vi "Edit IPI Dialog.vi"(8 "Coords":T1, 11 "Expr In":string) -> (3 "Expr Out":string)   [LabVIEW 2020]
uses:
  <vilib>/Utility/miscctls.llb/LVPoint32TypeDef.ctl
  epl-vi-lib/Utility VIs/Error Handling VIs/Error-Library Action.ctl
panel:
  in  "Tab Control":enum32{"Hist", "Error"}(tab)
  out "histogram":cluster{"X/1000":dbl[], "Y":dbl[]}(graph)
  out "Message":string
  out "replot":bool
  in  "Expr":string
  in  "Cancel":bool
  in  "OK":bool
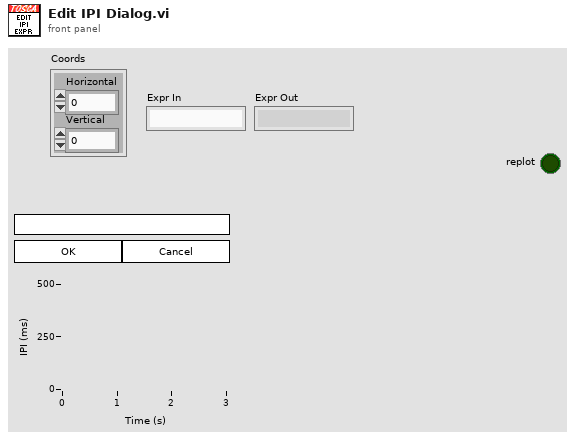
[diagram p1: front panel]
types:
  T1 = typedef "LVPoint32TypeDef.ctl" = cluster{"Horizontal":i32, "Vertical":i32}
  T2 = typedef "Error-Library Action.ctl" = enum16{"NONE", "Register", "Read"}
  T3 = typedef "Error Description.ctl" = cluster{"Code":i32, "Description":string, "Details":string}
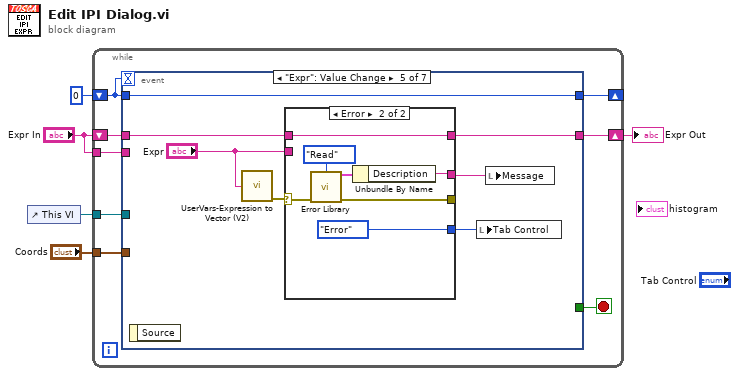
[diagram p0: block diagram]
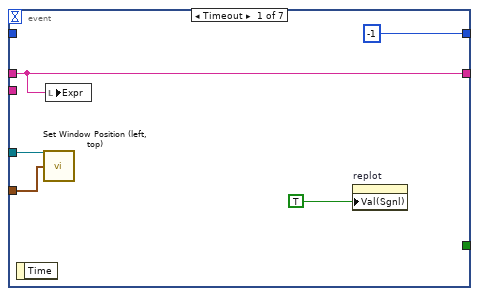
[diagram p2: hidden frame]
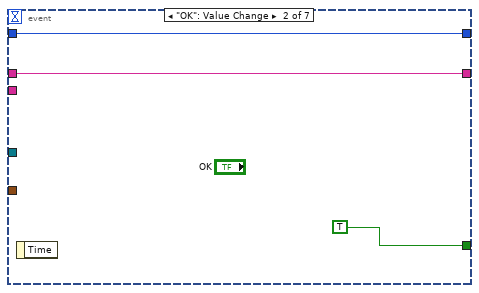
[diagram p3: hidden frame]
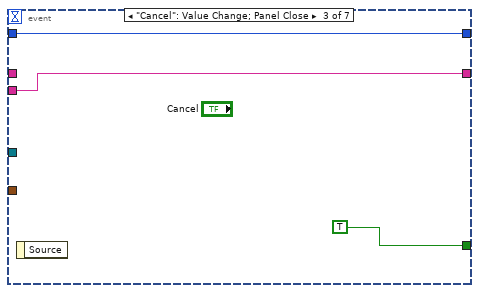
[diagram p4: hidden frame]
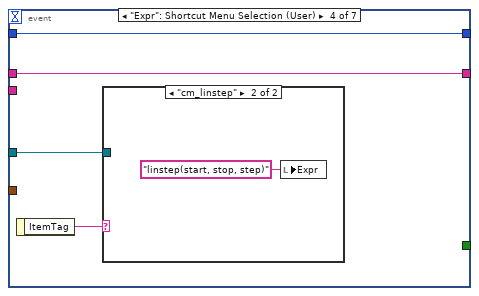
[diagram p5: hidden frame]
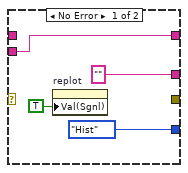
[diagram p7: hidden frame]
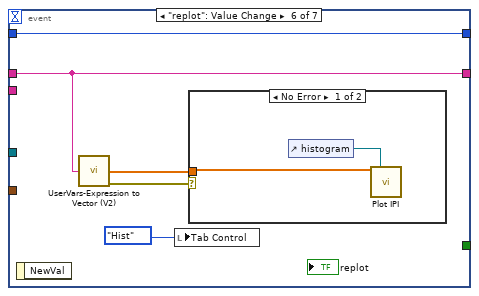
[diagram p8: hidden frame]
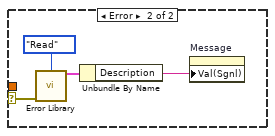
[diagram p9: hidden frame]
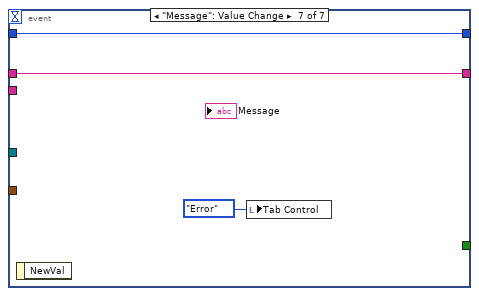
[diagram p10: hidden frame]
diagram:
  n1 = control-ref of="This VI"() -> (w1:refnum<vi>)
  n2 = while {
    shift-right: [w12] -> w5
    shift-left: "Expr In" -> [w13]
    shift-right: [w10] -> _
    shift-left: 0 -> [w9]
    tunnel: "Expr In" -> [w8]
    tunnel: "Coords" -> [w7]
    tunnel: w1 -> [w6]
    stop <- w11 stop-if-true
    n3 = event shown="[4] \"Expr\": Value Change" {
      selector: _ -> [_ _ _ _ _ _ _]
      dyn-events: _ -> [_ _ _ _ _ _ _]
      timeout: w9 -> [_ _ _ _ _ _ _]
      tunnel: w13 -> [w14 w19 _ w28 w35 w50 w61]
      tunnel: [w14 w19 w22 w28 w34 w50 w61] -> w12
      tunnel: [_ TRUE TRUE _ _ _ _] -> w11
      tunnel: w9 -> [_ w20 w23 w27 w36 w52 w60]
      tunnel: [-1 w20 w23 w27 w36 w52 w60] -> w10
      tunnel: w8 -> [_ _ w22 _ _ _ _]
      tunnel: w7 -> [w17 _ _ _ _ _ _]
      tunnel: w6 -> [w15 _ _ w26 _ _ _]
      event Timeout {
        n4 = event-data() -> ()  [unwired: 1 in, 1 out]
        n5 = call "Set Window Position (left, top).vi"("VI in"=w15, "Coords"=w17) -> ()  [unwired: 12 in, 2 out]
        n6 = local write "Expr"(w14) -> ()
        n7 = property on="replot" class="Bool (strict)"("Val(Sgnl)"=TRUE ("Value (Signaling)")) -> ()  [unwired: 2 in, 2 out]
      }
      event "OK": Value Change {
        n8 = event-data() -> ()  [unwired: 1 in, 1 out]
      }
      event "Cancel": Value Change; Panel Close {
        n9 = event-data() -> ()  [unwired: 1 in, 1 out]
      }
      event "Expr": Shortcut Menu Selection (User) {
        n10 = event-data() -> ("ItemTag"=w25:string)  [unwired: 1 in]
        n11 = case shown="\"cm_linstep\"" w25 {
          tunnel: w26 -> [_ _]
          frame "False", Default {
          }
          frame "cm_linstep" {
            n12 = local write "Expr"("linstep(start, stop, step)" ("Expr")) -> ()
          }
        }
      }
      event "Expr": Value Change {
        n13 = event-data() -> ()  [unwired: 1 in, 1 out]
        n14 = call "UserVars-Expression to Vector (V2).vi"("Expr"="Expr") -> ("error out"=w30:errorcluster)  [unwired: 13 in, 1 out]
        n15 = case shown="Error" w30 {
          selector: w30 -> [_ w46]
          tunnel: w35 -> [_ w47]
          tunnel: [w37 w47] -> w34
          tunnel: "Expr" -> [w37 _]
          tunnel: ["" ("Description") w42] -> w32
          tunnel: [_ w44] -> _
          tunnel: [enum32{"Hist", "Error"}."Hist" ("Tab Control") enum32{"Hist", "Error"}."Error" ("Tab Control")] -> w33
          frame No Error {
            n16 = property on="replot" class="Bool (strict)"("Val(Sgnl)"=TRUE ("Value (Signaling)")) -> ()  [unwired: 2 in, 2 out]
          }
          frame Error {
            n17 = call "Error Library.vi"("action"=Error-Library_Action."Read", "error in"=w46) -> ("Entry"=w43:T3, "error thru"=w44:errorcluster)  [unwired: 11 in, 1 out]
            n18 = Unbundle By Name(w43) -> ("Description"=w42:string)
          }
        }
        n19 = local write "Tab Control"(w33) -> ()
        n20 = local write "Message"(w32) -> ()
      }
      event "replot": Value Change {
        n21 = event-data() -> ()  [unwired: 1 in, 1 out]
        n22 = call "UserVars-Expression to Vector (V2).vi"("Expr"=w50) -> ("Values"=w49:dbl[], "error out"=w48:errorcluster)  [unwired: 13 in]
        n23 = local write "Tab Control"(enum32{"Hist", "Error"}."Hist" ("Tab Control")) -> ()
        n24 = case shown="No Error" w48 {
          selector: w48 -> [_ w58]
          tunnel: w49 -> [w54 _]
          frame No Error {
            n25 = control-ref of="histogram"() -> (w53:refnum<vi>)
            n26 = call "Plot IPI.vi"("Y"=w54, "XYGraph"=w53) -> ()  [unwired: 14 in]
          }
          frame Error {
            n27 = call "Error Library.vi"("action"=Error-Library_Action."Read", "error in"=w58) -> ("Entry"=w55:T3)  [unwired: 11 in, 2 out]
            n28 = Unbundle By Name(w55) -> ("Description"=w56:string)
            n29 = property on="Message" class="Str"("Val(Sgnl)"=w56) -> ()  [unwired: 2 in, 2 out]
          }
        }
      }
      event "Message": Value Change {
        n30 = event-data() -> ()  [unwired: 1 in, 1 out]
        n31 = local write "Tab Control"(enum32{"Hist", "Error"}."Error" ("Tab Control")) -> ()
      }
    }
  }
  "Expr Out" <- w5
